vi "Write File.vi"(8 "error in (no error)":errorcluster, 11 "Data.DAT in":refnum<class "Data.DAT.lvclass">) -> (0 "error out":errorcluster, 3 "Data.DAT out":refnum<class "Data.DAT.lvclass">)   [LabVIEW 2016, in "Data.DAT.lvclass"]
uses:
  Data.DAT.lvclass
  C:/user/patrick/git/LV-to-ITX/src/Data/Data.lvclass
  Data/Data.lvclass/Data.ctl
  Write DAT (2D).vi
  Data/Data.lvclass
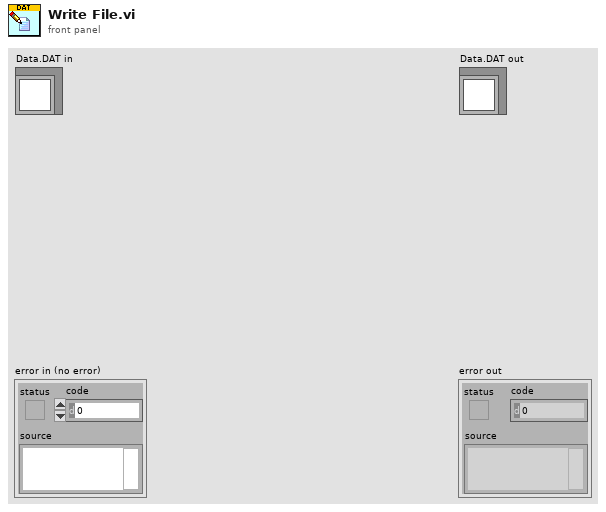
[diagram p1: front panel]
types:
  T1 = typedef "Data.lvclass/Dictionary--cluster.ctl" = cluster{"key":string, "value":variant}
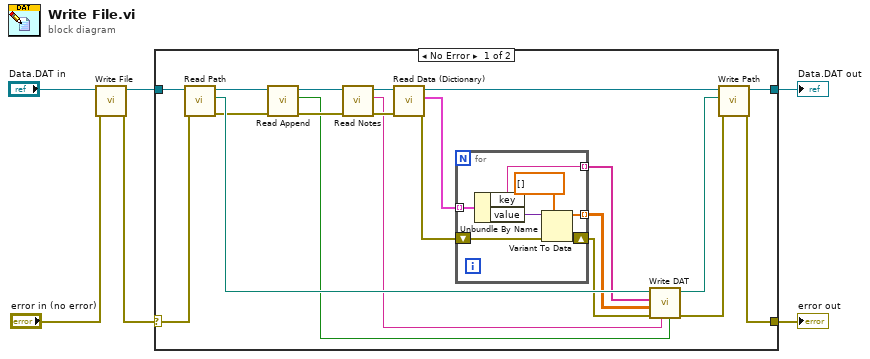
[diagram p0: block diagram]
diagram:
  n1 = call-parent "Write File.vi"("error in (no error)"="error in (no error)", "Data in"="Data.DAT in") -> ("error out"=w2:errorcluster, "Data out"=w4:refnum<class "Data.DAT.lvclass">)  [unwired: 8 in]
  n2 = case shown="No Error" w2 {
    selector: w2 -> [w24 w36]
    tunnel: [w18 w36] -> w5
    tunnel: w4 -> [w25 w35]
    tunnel: [w20 w35] -> w1
    frame No Error {
      n3 = call "Read Path.vi"("error in (no error)"=w24, "Data Save"=w25) -> ("error out"=w10:errorcluster, "Path"=w23:path, "Data Save out"=w11:refnum<class "Data.DAT.lvclass">)  [unwired: 7 in]
      n4 = call "Read Append.vi"("error in (no error)"=w10, "Data in"=w11) -> ("error out"=w8:errorcluster, "Append"=w7:bool, "Data out"=w9:refnum<class "Data.DAT.lvclass">)  [unwired: 7 in]
      n5 = call "Read Notes.vi"("error in (no error)"=w8, "Data Save"=w9) -> ("error out"=w26:errorcluster, "Comments"=w17:string, "Data Save out"=w27:refnum<class "Data.DAT.lvclass">)  [unwired: 7 in]
      n6 = call "Read Data (Dictionary).vi"("error in (no error)"=w26, "Data Save"=w27) -> ("error out"=w15:errorcluster, "Data (Dictionary)"=w16:T1[], "Data Save out"=w21:refnum<class "Data.DAT.lvclass">)  [unwired: 7 in]
      n7 = for {
        tunnel: w16 -> [w34] mode=indexing
        tunnel: [w29] -> w12 mode=indexing
        tunnel: [w28] -> w13 mode=indexing
        shift-right: [w31] -> w14
        shift-left: w15 -> [w32]
        n8 = Unbundle By Name(w34) -> ("key"=w29:string, "value"=w33:variant)
        n9 = Variant To Data(error in=w32, type=dbl[] [] ("Data"), Variant=w33) -> (data=w28:dbl[], error out=w31:errorcluster)
      }
      n10 = call-poly "Write DAT.vi"("append to file? (new file:F)"=w7, "Comments"=w17, "error in"=w14, "Data"=w13, "Headers"=w12, "path"=w23) -> ("error out"=w19:errorcluster, "new file path"=w22:path)  [unwired: 4 in]
      n11 = call "Write Path.vi"("error in (no error)"=w19, "Path"=w22, "Data Save"=w21) -> ("error out"=w18:errorcluster, "Data Save out"=w20:refnum<class "Data.DAT.lvclass">)  [unwired: 7 in]
    }
    frame Error {
    }
  }
  "error out" <- w5
  "Data.DAT out" <- w1
